vi "Create or Replace File.vi"(8 "error in":errorcluster, 10 "Log File Base Path":path) -> (0 "error out":errorcluster, 2 "File Path":path, 3 "Text refnum":refnum<file>)   [LabVIEW 2016, in "Logger.lvlib"]
doc: "_____\nBased on DQMH Project Template 6.1.0.94."
uses:
  Logger.lvlib
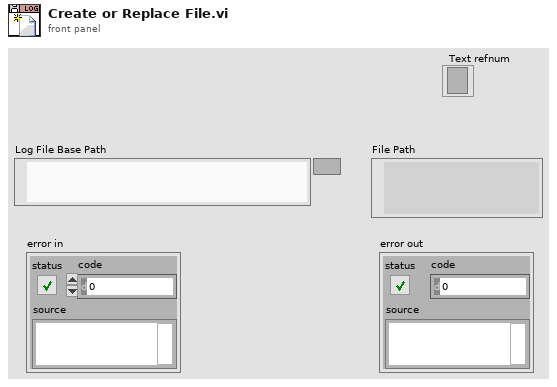
[diagram p1: front panel]
types:
  T1 = enum16{"open", "replace", "create", "open or create", "replace or create", "replace or create with confirmation"}
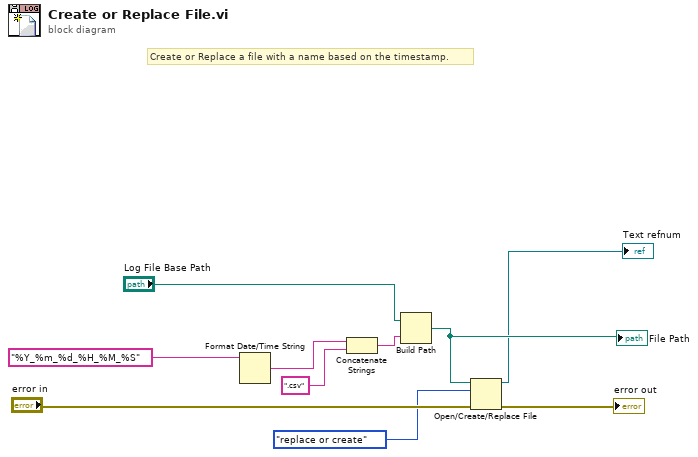
[diagram p0: block diagram]
diagram:
  # "Create or Replace a file with a name based on the timestamp."
  n1 = Format Date/Time String(time format string (%c)="%Y_%m_%d_%H_%M_%S") -> (date/time string=w4:string)  [unwired: 2 in]
  n2 = Concatenate Strings(w4, ".csv" ("string")) -> (w2:string)
  n3 = Build Path(base path="Log File Base Path", name or relative path=w2) -> (appended path=w7:path)
  "File Path" <- w7
  n4 = Open/Create/Replace File(file path (use dialog)=w7, error in="error in", operation (0:open)=T1."replace or create") -> (refnum out=→"Text refnum":refnum<file>, error out=→"error out":errorcluster)  [unwired: 3 in, 1 out]
